vi "Periodic Tasks.vi"(8 "error in":errorcluster) -> ()   [LabVIEW 2015]
doc: "This VI runs in parallel to other tasks. It can contain as many user-defined periodic loops as you need. These can carry out PID or other sorts of timed response."
uses:
  <vilib>/Rock Robotics/WPI/Utilities/WPI_GetSetVariantRefNum.vi
  <vilib>/Rock Robotics/Network Tables/NT Write Number.vi
  C:/Users/12ALEXANDER.TIETSORT/Downloads/ADIS16448-RoboRIO-Driver-master (1)/ADIS16448-RoboRIO-Driver-master/LabVIEW/ADI MXP IMU/FRC ADI MXP IMU.lvlib
panel:
  out "Sensor Ready?":bool
  out "IMU AHRS 2":cluster{"Pitch":dbl, "Roll":dbl, "Yaw":dbl}
  in  "Reset Angles?":bool
  out "Device Found?":bool
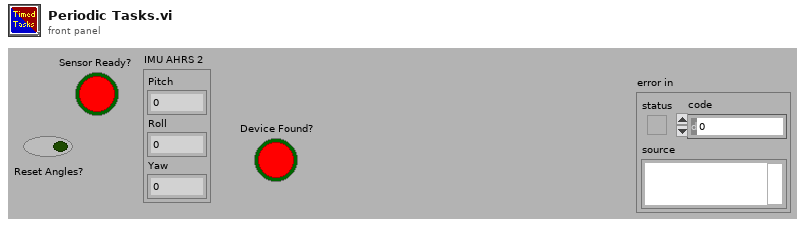
[diagram p1: front panel]
types:
  T1 = typedef "WPI_JoystickDevRef.ctl" = cluster{"Device":T2}
  T2 = typedef "WPI_JoystickDeviceEnum.ctl" = enum16{"USB 0", "USB 1", "USB 2", "USB 3", "USB 4", "USB 5"}
  T3 = typedef "WPI_RobotDriveDevRef.ctl" = cluster{"DevStatus":errorcluster, "Motors[]":T4[], "Square Inputs":bool, "Max Output":dbl}
  T4 = typedef "WPI_MotorControlDeviceRef.ctl" = cluster{"DeviceStatus":errorcluster, "Type":T5, "PWM":cluster{"PWM Channel":T6, "DeadBand":T7}, "CAN":cluster{"Device Number":u8, "Control Mode":T8, "Semaphore":T9, "Max Vout":dbl, "TalonSRX Control Mode":T10}, "Invert":bool}
  T5 = typedef "WPI_MotorControlType.ctl" = enum16{"PWM", "CAN", "CANTalonSRX"}
  T6 = typedef "FPGA_DIOPWMChannel.ctl" = enum8{"PWM 0", "PWM 1", "PWM 2", "PWM 3", "PWM 4", "PWM 5", "PWM 6", "PWM 7", "PWM 8", "PWM 9", "PWM MXP 0", "PWM MXP 1", "PWM MXP 2", "PWM MXP 3", "PWM MXP 4", "PWM MXP 5", "PWM MXP 6", "PWM MXP 7", "PWM MXP 8", "PWM MXP 9", "Invalid"}
  T7 = typedef "WPI_PWMDeadband.ctl" = cluster{"Name":string, "maxPositivePwm":i32, "minPositivePwm":i32, "centerPwm":i32, "maxNegativePwm":i32, "minNegativePwm":i32, "angularRange":u16}
  T8 = typedef "WPI_CANJaguar_ControlMode.ctl" = enum8{"Percent VBus", "Current", "Speed", "Position", "Voltage"}
  T9 = typedef "Semaphore RefNum" = refnum<k1>
  T10 = typedef "WPI_CANTalonSRX_APIControlMode.ctl" = enum8{"Percent VBus", "Speed", "Position", "Slave", "Unchanged / Invalid", "Voltage Compensation", "Current", "Motion Profile"}
  T11 = cluster{"JoystickDevRef":T1, "RobotDriveDevRef":T3}
  T12 = typedef "WPI_GyroDevRef.ctl" = cluster{"DevStatus":errorcluster, "Analog Channel":T13, "Offset":dbl, "Gain (VoltsPerDegree/Second)":dbl, "Gyro Type":enum16{"Analog", "XRS450"}, "Handle":i32, "SPI Bus":T14, "Device Found":bool, "Sample Rate":dbl, "Calibrate On Open":bool}
  T13 = typedef "FPGA_AIChannel.ctl" = enum8{"AI 0", "AI 1", "AI 2", "AI 3", "AI MXP 0", "AI MXP 1", "AI MXP 2", "AI MXP 3", "Invalid"}
  T14 = typedef "spi_bus.ctl" = enum16{"SPI On-Board, CS0", "SPI On-Board, CS1", "SPI On-Board, CS2", "SPI On-Board, CS3", "SPI MXP", "Invalid"}
  T15 = typedef "WPI_AnalogChannelDevRef.ctl" = cluster{"DevStatus":errorcluster, "Analog Channel":T13}
  T16 = typedef "FRC ADI MXP IMU.lvlib/WPI_AnalogDevicesIMUInterruptDevRef.ctl" = cluster{"SimpleGyroDevRef":T17, "InterruptRef":T18}
  T17 = typedef "FRC ADI MXP IMU.lvlib/WPI_AnalogDevicesIMUDevRef.ctl" = cluster{"DevStatus":errorcluster, "Handle":i32, "SPI Bus":T14, "Device Found":bool, "Sample Rate":dbl, "Device Ready":bool, "Yaw Axis":enum16{"X", "Y", "Z"}}
  T18 = typedef "WPI_InterruptRef.ctl" = cluster{"DevStatus":errorcluster, "InterruptIndex":T19}
  T19 = typedef "FPGA_InterruptIndex.ctl" = enum8{"0", "1", "2", "3", "4", "5", "6", "7", "Invalid"}
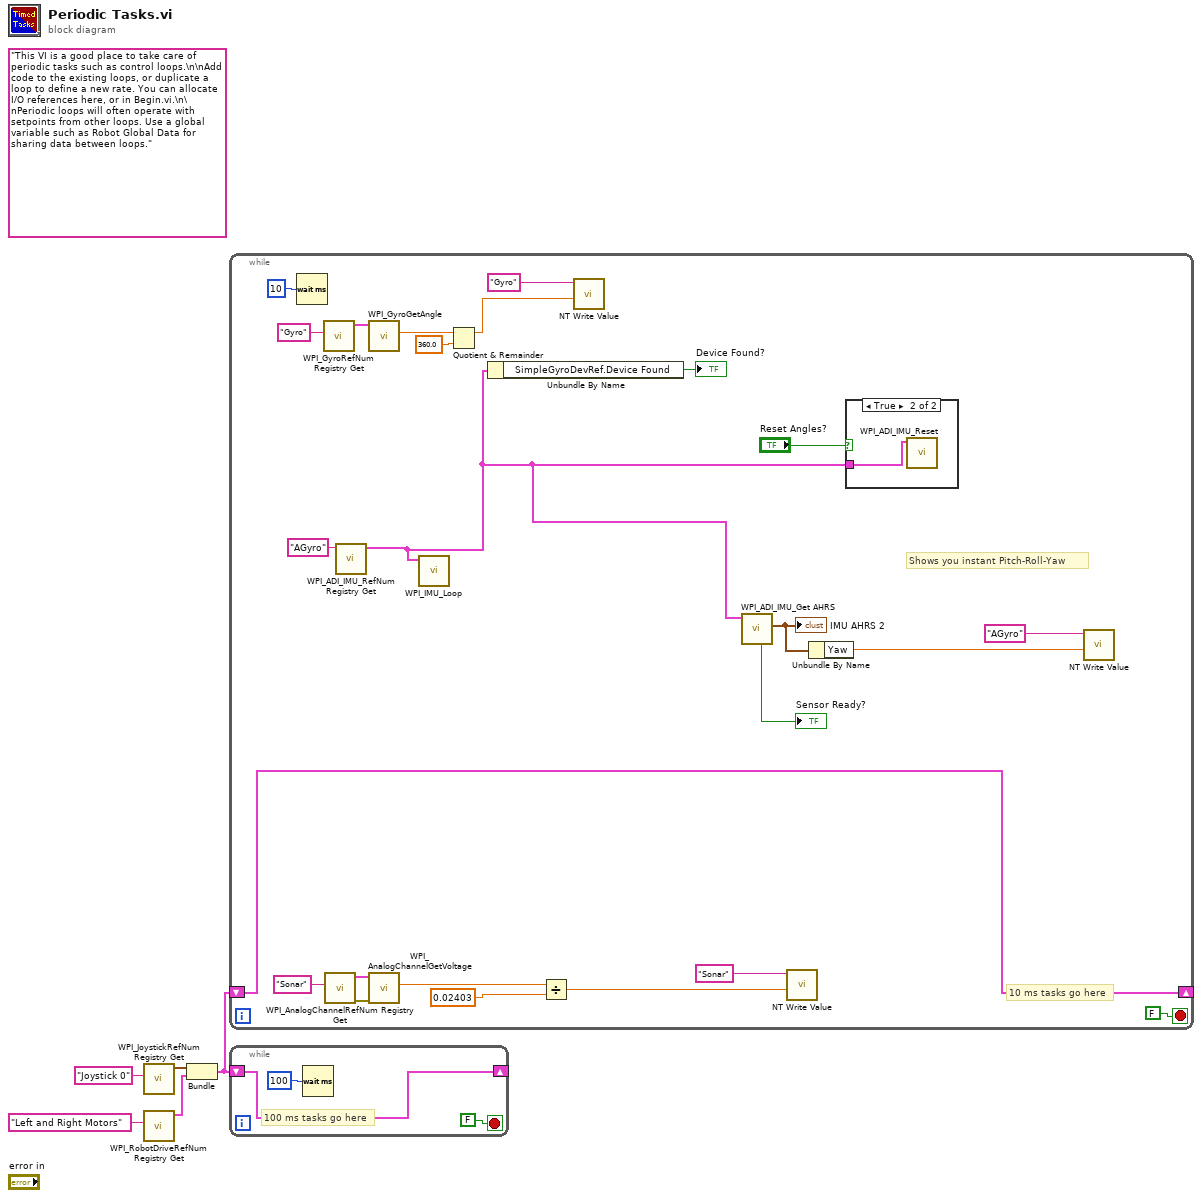
[diagram p0: block diagram]
diagram:
  (unwired) "This VI is a good place to take care of periodic tasks such as control loops.\n\nAdd code to the existing loops, or duplicate a loop to define a new rate. You can allocate I/O references here, or in Begin.vi.\n\nPeriodic loops will often operate with setpoints from other loops. Use a global variable such as Robot Global Data for sharing data between loops."
  n1 = call <vilib>:"WPI_JoystickRefNum Registry Get.vi"("refnum name"="Joystick 0") -> ("JoystickDevRef"=w3:T1)  [unwired: 1 in, 9 out]
  n2 = call <vilib>:"WPI_RobotDriveRefNum Registry Get.vi"("refnum name"="Left and Right Motors") -> ("RobotDriveDevRef"=w2:T3)  [unwired: 1 in, 9 out]
  n3 = Bundle("JoystickDevRef"=w3, "RobotDriveDevRef"=w2) -> (w1:T11)  [unwired: 1 out]
  n4 = while {
    shift-right: [w27] -> _
    shift-left: w1 -> [w27]
    stop <- FALSE stop-if-true
    # "Shows you instant Pitch-Roll-Yaw"
    # "10 ms tasks go here"
    n5 = Wait (ms)(milliseconds to wait=u32 10) -> ()  [unwired: 1 out]
    n6 = call <vilib>:"WPI_GyroRefNum Registry Get.vi"("refnum name"="Gyro") -> ("GyroDevRef"=w16:T12)  [unwired: 9 in, 1 out]
    n7 = call <vilib>:"WPI_AnalogChannelRefNum Registry Get.vi"("refnum name"="Sonar") -> ("error out"=w24:errorcluster, "AIDeviceRef"=w23:T15)  [unwired: 9 in]
    n8 = call "WPI_ADI_IMU_RefNum Registry Get.vi"("refnum name"="AGyro") -> ("ADI IMU Interrupt DevRef"=w6:T16)  [unwired: 9 in, 1 out]
    n9 = call <vilib>:"WPI_GyroGetAngle.vi"("GyroDevRef"=w16) -> ("Angle"=w19:dbl)  [unwired: 1 in, 9 out]
    n10 = call <vilib>:"WPI_AnalogChannelGetVoltage.vi"("error in (no error)"=w24, "AIDeviceRef"=w23) -> ("Voltage"=w22:dbl)  [unwired: 7 in, 2 out]
    n11 = call "WPI_IMU_Loop.vi"("ADI IMU Interrupt DevRef"=w6) -> ()  [unwired: 10 in, 1 out]
    n12 = Quotient & Remainder(x=w19, y=360.0) -> (x-y*floor(x/y)=w15:dbl)  [unwired: 1 out]
    n13 = Unbundle By Name(w6) -> ("SimpleGyroDevRef.Device Found"=→"Device Found?":bool)
    n14 = Divide(x=w22, y=0.02403) -> (x/y=w20:dbl)
    n15 = call-poly <vilib>:"NT Write Value.vi"("Numeric"=w15, "Name"="Gyro") -> ()  [unwired: 9 in, 1 out]
    n16 = call "WPI_ADI_IMU_Get AHRS.vi"("ADI IMU Interrupt DevRef"=w6) -> ("IMU AHRS"=w8:cluster{"Pitch":dbl, "Roll":dbl, "Yaw":dbl}, "Sensor Ready Out"=→"Sensor Ready?":bool)  [unwired: 6 in, 3 out]
    "IMU AHRS 2" <- w8
    n17 = call-poly <vilib>:"NT Write Value.vi"("Numeric"=w20, "Name"="Sonar") -> ()  [unwired: 9 in, 1 out]
    n18 = Unbundle By Name(w8) -> ("Yaw"=w9:dbl)
    n19 = case shown="True" "Reset Angles?" {
      tunnel: w6 -> [_ w30]
      frame False {
      }
      frame True {
        n20 = call "WPI_ADI_IMU_Reset.vi"("ADI IMU Interrupt DevRef"=w30) -> ()  [unwired: 9 in, 2 out]
      }
    }
    n21 = call-poly <vilib>:"NT Write Value.vi"("Numeric"=w9, "Name"="AGyro") -> ()  [unwired: 9 in, 1 out]
  }
  n22 = while {
    shift-right: [w31] -> _
    shift-left: w1 -> [w31]
    stop <- FALSE stop-if-true
    # "100 ms tasks go here"
    n23 = Wait (ms)(milliseconds to wait=u32 100) -> ()  [unwired: 1 out]
  }
